vi "Time.UTC - Local Time Diff.vi"(11 "LocalTime":timestamp) -> (2 "Time Diff":dbl, 3 "UTC":timestamp)   [LabVIEW 2019]
panel:
  out "Local":timestamp
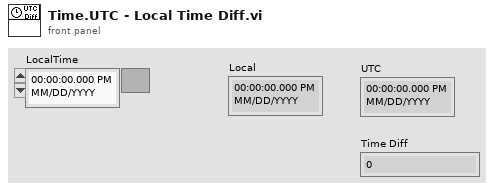
[diagram p1: front panel]
types:
  T1 = typedef "LVDateTimeRec.ctl" = cluster{"fractional second":dbl, "second":i32, "minute":i32, "hour":i32, "day of month":i32, "month":i32, "year":i32, "day of week":i32, "day of year":i32, "DST":i32}
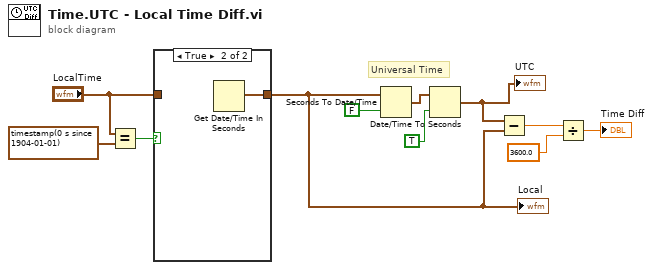
[diagram p0: block diagram]
diagram:
  # "Universal Time"
  n1 = Equal?(x="LocalTime", y=timestamp(0 s since 1904-01-01)) -> (x = y?=w10:bool)
  n2 = case shown="True" w10 {
    tunnel: "LocalTime" -> [w12 _]
    tunnel: [w12 w13] -> w3
    frame False {
    }
    frame True {
      n3 = Get Date/Time In Seconds() -> (seconds since 1Jan1904=w13:timestamp)
    }
  }
  "Local" <- w3
  n4 = Seconds To Date/Time(time stamp (now)=w3, to UTC (F)=FALSE) -> (date time rec=w9:T1)
  n5 = Date/Time To Seconds(1:TRUE ("to UTC (F)"), 2:w9) -> (0:w4:timestamp)
  "UTC" <- w4
  n6 = Subtract(x=w4, y=w3) -> (x-y=w8:dbl)
  n7 = Divide(x=w8, y=3600.0) -> (x/y=→"Time Diff":dbl)
